vi "Teaching.vi"() -> ()   [LabVIEW 2014]
panel:
  out "?":string
  out "?":string
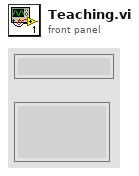
[diagram p1: front panel]
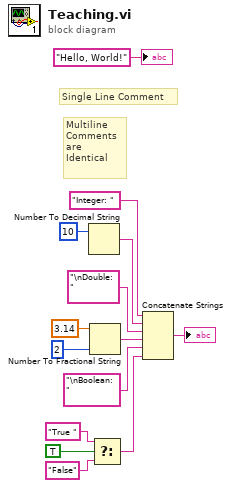
[diagram p0: block diagram]
diagram:
  # "Multiline\nComments\nare\nIdentical"
  # "Single Line Comment"
  n1 = Number To Decimal String(number=10) -> (decimal integer string=w12:string)  [unwired: 1 in]
  n2 = Number To Fractional String(number=3.14, precision (6)=i16 2) -> (F-format string=w1:string)  [unwired: 2 in]
  n3 = Select(t="True " ("string"), s=TRUE, f="False") -> (s? t:f=w4:string)
  n4 = Concatenate Strings("Integer: ", w12, "\nDouble: " ("string"), w1, "\nBoolean: " ("string"), w4) -> (→"?":string)
  "?" <- "Hello, World!"
